vi "双通道示波器.vi"() -> ()   [LabVIEW 2022 SP3]
uses:
  <vilib>/Analysis/3filter.llb/Butterworth Filter (DBL).vi
  <vilib>/measure/matone.llb/Extract Single Tone Information 1 Chan.vi
  <vilib>/measure/NI_MABase.lvlib
  <vilib>/measure/NI_MAPro.lvlib
  <vilib>/Analysis/NI_AALBase.lvlib
panel:
  in  "选项卡控件":enum32{"基本参数", "滤波"}(tab)
  in  "CH0幅值单位调节":dbl(knob) scale=1.0..2.0
  in  "CH0幅值偏移":dbl(knob) scale=0.0..10.0
  in  "CH0":bool
  in  "CH1幅值单位调节":dbl(knob) scale=1.0..2.0
  in  "CH1幅值偏移":dbl(knob) scale=0.0..10.0
  in  "CH1":bool
  in  "CH1采样频率":i16(slide) scale=0.0..100.0
  in  "CH0采样频率":i16(slide) scale=0.0..100.0
  in  "CH0低截止频率":i16(slide) scale=0.0..5.0
  in  "CH0高截止频率":i16(slide) scale=0.0..5.0
  in  "CH0滤波器阶数":u8
  in  "CH1滤波器阶数":u8
  in  "CH1低截止频率":i16(slide) scale=0.0..5.0
  in  "CH1高截止频率":i16(slide) scale=0.0..10.0
  in  "CH1滤波器类型":u16(ring) items=["低通", "高通", "带通", "带阻"]
  in  "CH1滤波开关":bool
  in  "CH0滤波器类型":u16(ring) items=["低通", "高通", "带通", "带阻"]
  in  "CH0滤波开关":bool
  out "波形图":dbl[][](graph)
  out "CH1频率":dbl
  out "CH0频率":dbl
  out "CH0幅值":dbl
  out "CH1幅值":dbl
  out "CH1指示灯":bool
  out "CH0指示灯":bool
  in  "扫描频率":dbl(knob) scale=0.0..5.0
  in  "示波器开关":bool
  out "通道2指示灯":bool
  out "通道1指示灯":bool
  in  "信号发生器开关":bool
  in  "通道二开关":bool
  in  "通道一开关":bool
  in  "通道2自定义公式":string
  in  "通道2波形类型":u16(ring) items=["三角波", "正弦波", "自定义波形", "方波", "锯齿波"]
  out "通道2波形图表":waveform(dbl)(graph)
  in  "通道2偏移量":i64(knob) scale=-5.0..5.0
  in  "通道2标准差":dbl(knob) scale=0.0..1.0
  in  "通道2幅度":i64(knob) scale=0.0..10.0
  in  "通道2频率":dbl(knob) scale=0.0..1.0
  out "通道2波形信息":string
  out "通道1波形图表":waveform(dbl)(graph)
  out "通道1波形信息":string
  in  "通道1自定义公式":string
  in  "采样数":i64(slide) scale=1.0..5000.0
  in  "采样率":i64(slide) scale=150.0..1500.0
  in  "通道1偏移量":i64(knob) scale=-5.0..5.0
  in  "通道1标准差":dbl(knob) scale=0.0..1.0
  in  "通道1幅度":i64(knob) scale=0.0..10.0
  in  "通道1频率":dbl(knob) scale=0.0..1.0
  in  "通道1波形类型":u16(ring) items=["三角波", "正弦波", "自定义波形", "方波", "锯齿波"]
  # "信号发生器   MZ-0016"
  # "示波器  MZ-0016"
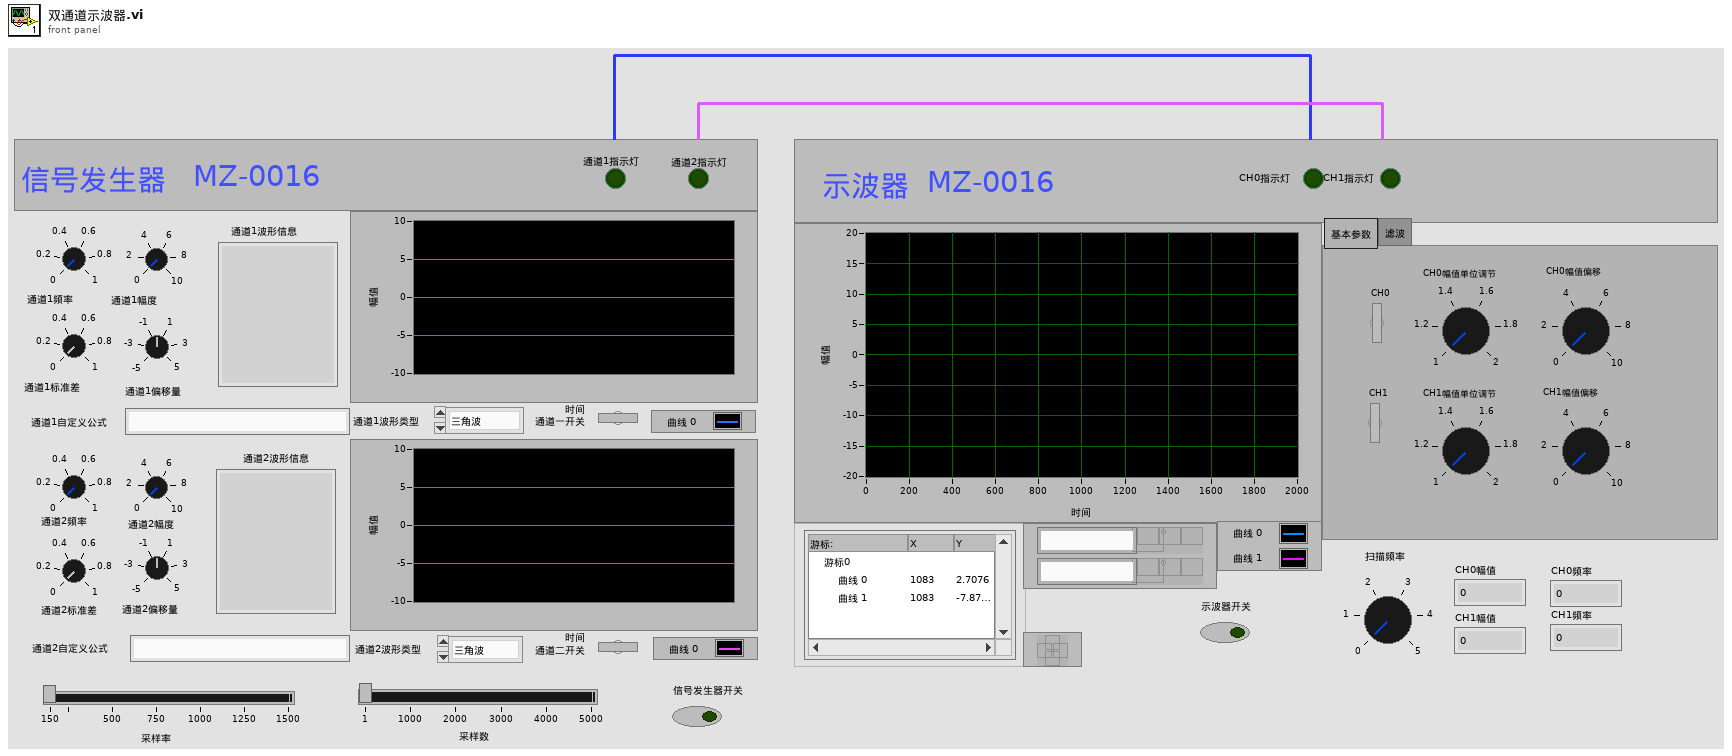
[diagram p1: front panel]
types:
  T1 = enum8{"Enabled", "Disabled", "Disabled and Grayed Out"}
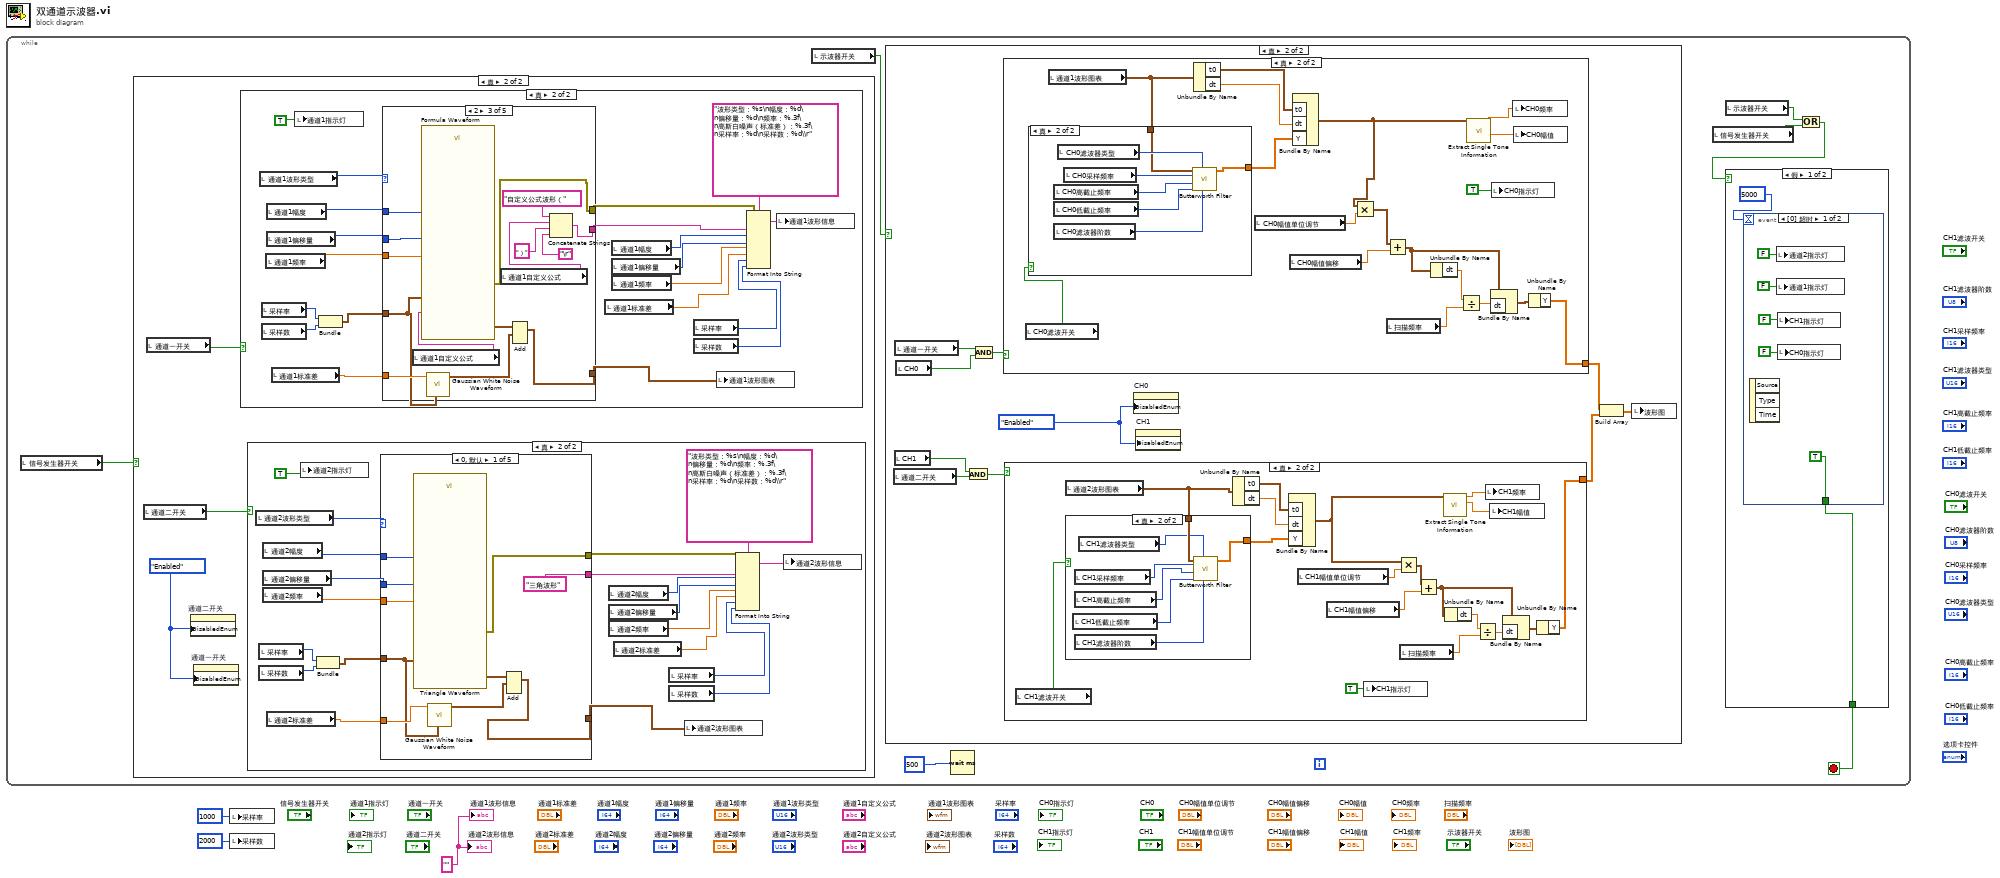
[diagram p0: block diagram]
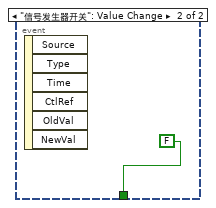
[diagram p2: hidden frame]
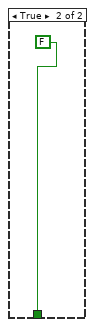
[diagram p3: hidden frame]
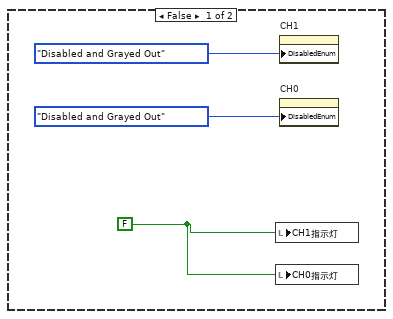
[diagram p4: hidden frame]
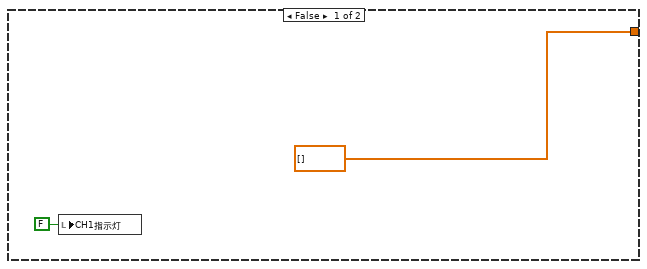
[diagram p5: hidden frame]
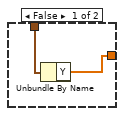
[diagram p6: hidden frame]
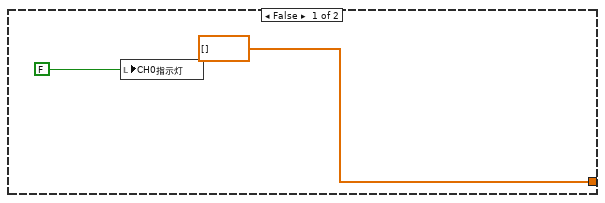
[diagram p7: hidden frame]
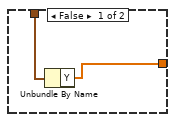
[diagram p8: hidden frame]
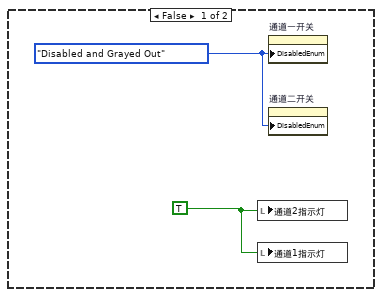
[diagram p9: hidden frame]
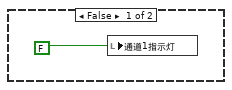
[diagram p10: hidden frame]
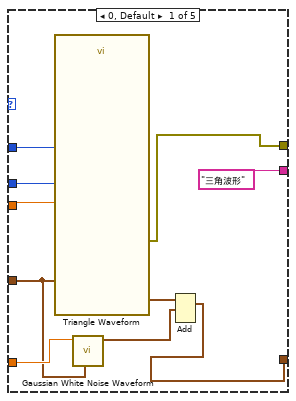
[diagram p11: hidden frame]
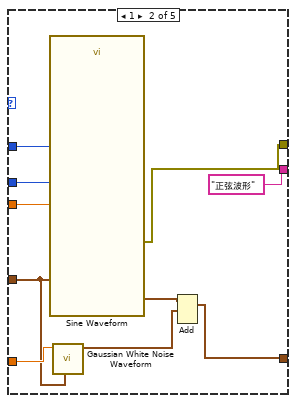
[diagram p12: hidden frame]
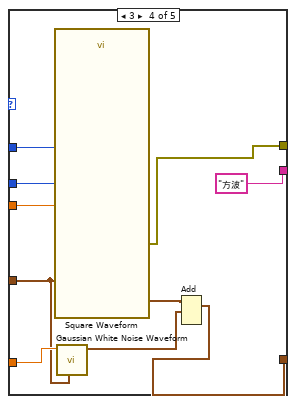
[diagram p13: hidden frame]
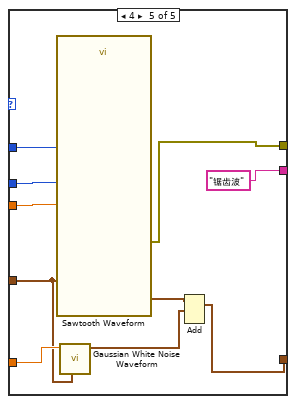
[diagram p14: hidden frame]
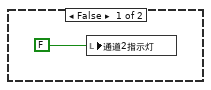
[diagram p15: hidden frame]
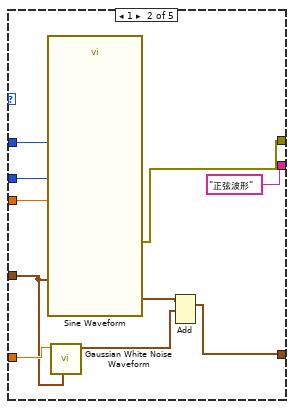
[diagram p16: hidden frame]
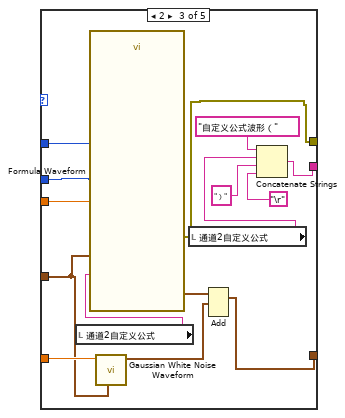
[diagram p17: hidden frame]
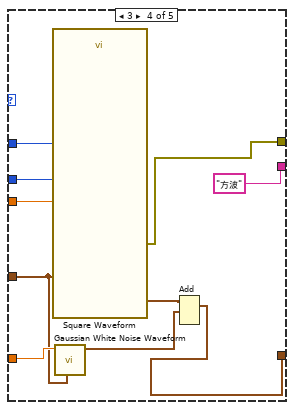
[diagram p18: hidden frame]
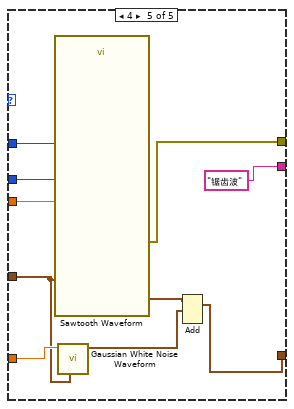
[diagram p19: hidden frame]
diagram:
  w3 = "" ("波形信息")
  n1 = while {
    stop <- w6 stop-if-true
    n2 = local read "信号发生器开关"() -> (w4:bool)
    n3 = case shown="真" w4 {
      frame False {
        w91 = T1."Disabled and Grayed Out" ("禁用")
        w92 = TRUE ("通道2指示灯")
        n4 = local write "通道2指示灯"(w92) -> ()
        n5 = local write "通道1指示灯"(w92) -> ()
        n6 = property on="通道一开关" class="Bool (严格)"("DisabledEnum"=w91) -> ()  [unwired: 2 in, 2 out]
        n7 = property on="通道二开关" class="Bool (严格)"("DisabledEnum"=w91) -> ()  [unwired: 2 in, 2 out]
      }
      frame True {
        w95 = T1."Enabled" ("禁用")
        n8 = local read "通道二开关"() -> (w93:bool)
        n9 = local read "通道一开关"() -> (w94:bool)
        n10 = property on="通道二开关" class="Bool (严格)"("DisabledEnum"=w95) -> ()  [unwired: 2 in, 2 out]
        n11 = property on="通道一开关" class="Bool (严格)"("DisabledEnum"=w95) -> ()  [unwired: 2 in, 2 out]
        n12 = case shown="真" w94 {
          frame False {
            n13 = local write "通道1指示灯"(FALSE ("通道1")) -> ()
          }
          frame True {
            n14 = local read "通道1波形类型"() -> (w116:u16)
            n15 = local read "采样率"() -> (w111:i64)
            n16 = local read "采样数"() -> (w110:i64)
            n17 = local read "通道1频率"() -> (w114:dbl)
            n18 = local read "通道1幅度"() -> (w112:i64)
            n19 = local read "通道1偏移量"() -> (w113:i64)
            n20 = local read "通道1标准差"() -> (w115:dbl)
            n21 = local write "通道1指示灯"(TRUE ("通道1")) -> ()
            n22 = Bundle("采样率"=w111, "采样数"=w110) -> (w109:cluster{"采样率":i64, "采样数":i64})  [unwired: 1 in]
            n23 = case shown="2" w116 {
              tunnel: w115 -> [w123 w133 w146 w155 w166]
              tunnel: w114 -> [w124 w134 w151 w158 w167]
              tunnel: w113 -> [w125 w135 w150 w157 w168]
              tunnel: w112 -> [w126 w136 w149 w156 w169]
              tunnel: w109 -> [w122 w132 w145 w154 w164]
              tunnel: [w119 w129 w139 w159 w165] -> w98
              tunnel: ["三角波形" "正弦波形" w138 "方波" "锯齿波"] -> w100
              tunnel: [w117 w127 w137 w152 w162] -> w99
              frame 0, Default {
                n24 = call <vilib>:"Triangle Waveform.vi"("offset"=w125, "sampling info"=w122, "amplitude"=w126, "frequency"=w124) -> ("error out"=w117:errorcluster, "signal out"=w121:waveform(dbl))  [unwired: 6 in]
                n25 = call <vilib>:"Gaussian White Noise Waveform.vi"("sampling info"=w122, "standard deviation"=w123) -> ("signal out"=w120:waveform(dbl))  [unwired: 8 in, 1 out]
                n26 = Add(1:w120, 2:w121) -> (0:w119:waveform(dbl))  [unwired: 1 in, 1 out]
              }
              frame 1 {
                n27 = call <vilib>:"Sine Waveform.vi"("offset"=w135, "sampling info"=w132, "amplitude"=w136, "frequency"=w134) -> ("error out"=w127:errorcluster, "signal out"=w131:waveform(dbl))  [unwired: 6 in]
                n28 = call <vilib>:"Gaussian White Noise Waveform.vi"("sampling info"=w132, "standard deviation"=w133) -> ("signal out"=w130:waveform(dbl))  [unwired: 8 in, 1 out]
                n29 = Add(1:w130, 2:w131) -> (0:w129:waveform(dbl))  [unwired: 1 in, 1 out]
              }
              frame 2 {
                n30 = local read "通道1自定义公式"() -> (w148:string)
                n31 = call <vilib>:"Formula Waveform.vi"("offset"=w150, "sampling info"=w145, "formula"=w148, "amplitude"=w149, "frequency"=w151) -> ("error out"=w137:errorcluster, "signal out"=w147:waveform(dbl))  [unwired: 5 in]
                n32 = call <vilib>:"Gaussian White Noise Waveform.vi"("sampling info"=w145, "standard deviation"=w146) -> ("signal out"=w144:waveform(dbl))  [unwired: 8 in, 1 out]
                n33 = local read "通道1自定义公式"() -> (w142:string)
                n34 = Add(1:w144, 2:w147) -> (0:w139:waveform(dbl))  [unwired: 1 in, 1 out]
                n35 = Concatenate Strings("自定义公式波形（", w142, "）" ("字符串"), "\r") -> (w138:string)
              }
              frame 3 {
                n36 = call <vilib>:"Square Waveform.vi"("offset"=w157, "sampling info"=w154, "amplitude"=w156, "frequency"=w158) -> ("error out"=w152:errorcluster, "signal out"=w161:waveform(dbl))  [unwired: 6 in]
                n37 = call <vilib>:"Gaussian White Noise Waveform.vi"("sampling info"=w154, "standard deviation"=w155) -> ("signal out"=w160:waveform(dbl))  [unwired: 8 in, 1 out]
                n38 = Add(1:w160, 2:w161) -> (0:w159:waveform(dbl))  [unwired: 1 in, 1 out]
              }
              frame 4 {
                n39 = call <vilib>:"Sawtooth Waveform.vi"("offset"=w168, "sampling info"=w164, "amplitude"=w169, "frequency"=w167) -> ("error out"=w162:errorcluster, "signal out"=w171:waveform(dbl))  [unwired: 6 in]
                n40 = call <vilib>:"Gaussian White Noise Waveform.vi"("sampling info"=w164, "standard deviation"=w166) -> ("signal out"=w170:waveform(dbl))  [unwired: 8 in, 1 out]
                n41 = Add(1:w170, 2:w171) -> (0:w165:waveform(dbl))  [unwired: 1 in, 1 out]
              }
            }
            n42 = local read "通道1标准差"() -> (w106:dbl)
            n43 = local read "通道1幅度"() -> (w103:i64)
            n44 = local read "通道1偏移量"() -> (w104:i64)
            n45 = local read "通道1频率"() -> (w105:dbl)
            n46 = local read "采样率"() -> (w107:i64)
            n47 = local read "采样数"() -> (w108:i64)
            n48 = local write "通道1波形图表"(w98) -> ()
            n49 = Format Into String(format string="波形类型：%s\n幅度：%d\n偏移量：%d\n频率：%.3f\n高斯白噪声（标准差）：%.3f\n采样率：%d\n采样数：%d\\r", error in=w99, w100, w103, w104, w105, w106, w107, w108) -> (resulting string=w101:string)  [unwired: 1 in, 1 out]
            n50 = local write "通道1波形信息"(w101) -> ()
          }
        }
        n51 = case shown="真" w93 {
          frame False {
            n52 = local write "通道2指示灯"(FALSE ("通道2")) -> ()
          }
          frame True {
            n53 = local read "通道2波形类型"() -> (w174:u16)
            n54 = local read "采样率"() -> (w179:i64)
            n55 = local read "采样数"() -> (w180:i64)
            n56 = local read "通道2幅度"() -> (w178:i64)
            n57 = local read "通道2偏移量"() -> (w177:i64)
            n58 = local read "通道2频率"() -> (w176:dbl)
            n59 = local read "通道2标准差"() -> (w175:dbl)
            n60 = local write "通道2指示灯"(TRUE ("通道2")) -> ()
            n61 = Bundle("采样率"=w179, "采样数"=w180) -> (w181:cluster{"采样率":i64, "采样数":i64})  [unwired: 1 in]
            n62 = case shown="0, 默认" w174 {
              tunnel: w175 -> [w199 w209 w222 w231 w242]
              tunnel: w176 -> [w200 w210 w227 w234 w243]
              tunnel: w177 -> [w201 w211 w226 w233 w244]
              tunnel: w178 -> [w202 w212 w225 w232 w245]
              tunnel: w181 -> [w198 w208 w221 w230 w240]
              tunnel: [w195 w205 w215 w235 w241] -> w192
              tunnel: ["三角波形" "正弦波形" w214 "方波" "锯齿波"] -> w190
              tunnel: [w193 w203 w213 w228 w238] -> w191
              frame 0, Default {
                n63 = call <vilib>:"Triangle Waveform.vi"("offset"=w201, "sampling info"=w198, "amplitude"=w202, "frequency"=w200) -> ("error out"=w193:errorcluster, "signal out"=w197:waveform(dbl))  [unwired: 6 in]
                n64 = call <vilib>:"Gaussian White Noise Waveform.vi"("sampling info"=w198, "standard deviation"=w199) -> ("signal out"=w196:waveform(dbl))  [unwired: 8 in, 1 out]
                n65 = Add(1:w196, 2:w197) -> (0:w195:waveform(dbl))  [unwired: 1 in, 1 out]
              }
              frame 1 {
                n66 = call <vilib>:"Sine Waveform.vi"("offset"=w211, "sampling info"=w208, "amplitude"=w212, "frequency"=w210) -> ("error out"=w203:errorcluster, "signal out"=w207:waveform(dbl))  [unwired: 6 in]
                n67 = call <vilib>:"Gaussian White Noise Waveform.vi"("sampling info"=w208, "standard deviation"=w209) -> ("signal out"=w206:waveform(dbl))  [unwired: 8 in, 1 out]
                n68 = Add(1:w206, 2:w207) -> (0:w205:waveform(dbl))  [unwired: 1 in, 1 out]
              }
              frame 2 {
                n69 = local read "通道2自定义公式"() -> (w224:string)
                n70 = call <vilib>:"Formula Waveform.vi"("offset"=w226, "sampling info"=w221, "formula"=w224, "amplitude"=w225, "frequency"=w227) -> ("error out"=w213:errorcluster, "signal out"=w223:waveform(dbl))  [unwired: 5 in]
                n71 = call <vilib>:"Gaussian White Noise Waveform.vi"("sampling info"=w221, "standard deviation"=w222) -> ("signal out"=w220:waveform(dbl))  [unwired: 8 in, 1 out]
                n72 = local read "通道2自定义公式"() -> (w218:string)
                n73 = Add(1:w220, 2:w223) -> (0:w215:waveform(dbl))  [unwired: 1 in, 1 out]
                n74 = Concatenate Strings("自定义公式波形（", w218, "）" ("字符串"), "\r") -> (w214:string)
              }
              frame 3 {
                n75 = call <vilib>:"Square Waveform.vi"("offset"=w233, "sampling info"=w230, "amplitude"=w232, "frequency"=w234) -> ("error out"=w228:errorcluster, "signal out"=w237:waveform(dbl))  [unwired: 6 in]
                n76 = call <vilib>:"Gaussian White Noise Waveform.vi"("sampling info"=w230, "standard deviation"=w231) -> ("signal out"=w236:waveform(dbl))  [unwired: 8 in, 1 out]
                n77 = Add(1:w236, 2:w237) -> (0:w235:waveform(dbl))  [unwired: 1 in, 1 out]
              }
              frame 4 {
                n78 = call <vilib>:"Sawtooth Waveform.vi"("offset"=w244, "sampling info"=w240, "amplitude"=w245, "frequency"=w243) -> ("error out"=w238:errorcluster, "signal out"=w247:waveform(dbl))  [unwired: 6 in]
                n79 = call <vilib>:"Gaussian White Noise Waveform.vi"("sampling info"=w240, "standard deviation"=w242) -> ("signal out"=w246:waveform(dbl))  [unwired: 8 in, 1 out]
                n80 = Add(1:w246, 2:w247) -> (0:w241:waveform(dbl))  [unwired: 1 in, 1 out]
              }
            }
            n81 = local read "通道2幅度"() -> (w187:i64)
            n82 = local read "通道2偏移量"() -> (w186:i64)
            n83 = local read "通道2频率"() -> (w185:dbl)
            n84 = local read "通道2标准差"() -> (w184:dbl)
            n85 = local read "采样率"() -> (w183:i64)
            n86 = local read "采样数"() -> (w182:i64)
            n87 = local write "通道2波形图表"(w192) -> ()
            n88 = Format Into String(format string="波形类型：%s\n幅度：%d\n偏移量：%d\n频率：%.3f\n高斯白噪声（标准差）：%.3f\n采样率：%d\n采样数：%d\\r", error in=w191, w190, w187, w186, w185, w184, w183, w182) -> (resulting string=w189:string)  [unwired: 1 in, 1 out]
            n89 = local write "通道2波形信息"(w189) -> ()
          }
        }
      }
    }
    n90 = local read "示波器开关"() -> (w9:bool)
    n91 = case shown="真" w9 {
      frame False {
        w20 = FALSE ("CH1指示灯")
        n92 = local write "CH1指示灯"(w20) -> ()
        n93 = local write "CH0指示灯"(w20) -> ()
        n94 = property on="CH1" class="Bool (严格)"("DisabledEnum"=T1."Disabled and Grayed Out" ("禁用")) -> ()  [unwired: 2 in, 2 out]
        n95 = property on="CH0" class="Bool (严格)"("DisabledEnum"=T1."Disabled and Grayed Out" ("禁用")) -> ()  [unwired: 2 in, 2 out]
      }
      frame True {
        w26 = T1."Enabled" ("禁用")
        n96 = local read "通道二开关"() -> (w30:bool)
        n97 = local read "CH1"() -> (w29:bool)
        n98 = local read "通道一开关"() -> (w32:bool)
        n99 = local read "CH0"() -> (w31:bool)
        n100 = And(x=w29, y=w30) -> (x .and. y?=w27:bool)
        n101 = And(x=w32, y=w31) -> (x .and. y?=w23:bool)
        n102 = case shown="真" w23 {
          tunnel: [dbl[] [] ("Y") w70] -> w25
          frame False {
            n103 = local write "CH0指示灯"(FALSE ("CH0指示灯")) -> ()
          }
          frame True {
            n104 = local read "CH0滤波开关"() -> (w64:bool)
            n105 = local read "通道1波形图表"() -> (w69:waveform(dbl))
            n106 = case shown="真" w64 {
              tunnel: w69 -> [w83 w89]
              tunnel: [w82 w84] -> w65
              frame False {
                n107 = Unbundle By Name(w83) -> ("Y"=w82:dbl[])
              }
              frame True {
                n108 = local read "CH0高截止频率"() -> (w87:i16)
                n109 = local read "CH0低截止频率"() -> (w86:i16)
                n110 = local read "CH0滤波器阶数"() -> (w85:u8)
                n111 = local read "CH0滤波器类型"() -> (w90:u16)
                n112 = local read "CH0采样频率"() -> (w88:i16)
                n113 = call-poly <vilib>:"Butterworth Filter.vi"("order"=w85, "filter type"=w90, "low cutoff freq: fl"=w86, "high cutoff freq: fh"=w87, "sampling freq: fs"=w88, "X"=w89) -> ("Filtered X"=w84:dbl[])  [unwired: 2 in, 1 out]
              }
            }
            n114 = Unbundle By Name(w69) -> ("t0"=w68:timestamp, "dt"=w67:dbl)
            n115 = local read "CH0幅值单位调节"() -> (w79:dbl)
            n116 = local read "CH0幅值偏移"() -> (w77:dbl)
            n117 = Bundle By Name("t0"=w68, "dt"=w67, "Y"=w65) -> (w66:waveform(dbl))  [unwired: 1 in]
            n118 = Multiply(x=w66, y=w79) -> (x*y=w78:waveform(dbl))
            n119 = Add(x=w78, y=w77) -> (x+y=w73:waveform(dbl))
            n120 = local read "扫描频率"() -> (w75:dbl)
            n121 = Unbundle By Name(w73) -> ("dt"=w76:dbl)
            n122 = Divide(x=w76, y=w75) -> (x/y=w74:dbl)
            n123 = call-poly <vilib>:"Extract Single Tone Information.vi"("time signal in"=w66) -> ("detected amplitude"=w80:dbl, "detected frequency"=w81:dbl)  [unwired: 5 in, 4 out]
            n124 = Bundle By Name(cluster=w73, "dt"=w74) -> (w72:waveform(dbl))
            n125 = local write "CH0指示灯"(TRUE ("CH0指示灯")) -> ()
            n126 = local write "CH0频率"(w81) -> ()
            n127 = local write "CH0幅值"(w80) -> ()
            n128 = Unbundle By Name(w72) -> ("Y"=w70:dbl[])
          }
        }
        n129 = case shown="真" w27 {
          tunnel: [dbl[] [] ("Y") w42] -> w24
          frame False {
            n130 = local write "CH1指示灯"(FALSE ("CH1指示灯")) -> ()
          }
          frame True {
            n131 = local read "CH1滤波开关"() -> (w35:bool)
            n132 = local read "通道2波形图表"() -> (w40:waveform(dbl))
            n133 = case shown="真" w35 {
              tunnel: w40 -> [w54 w61]
              tunnel: [w53 w60] -> w37
              frame False {
                n134 = Unbundle By Name(w54) -> ("Y"=w53:dbl[])
              }
              frame True {
                n135 = local read "CH1低截止频率"() -> (w56:i16)
                n136 = local read "CH1采样频率"() -> (w58:i16)
                n137 = local read "CH1高截止频率"() -> (w57:i16)
                n138 = local read "CH1滤波器阶数"() -> (w55:u8)
                n139 = local read "CH1滤波器类型"() -> (w59:u16)
                n140 = call-poly <vilib>:"Butterworth Filter.vi"("order"=w55, "filter type"=w59, "low cutoff freq: fl"=w56, "high cutoff freq: fh"=w57, "sampling freq: fs"=w58, "X"=w61) -> ("Filtered X"=w60:dbl[])  [unwired: 2 in, 1 out]
              }
            }
            n141 = Unbundle By Name(w40) -> ("t0"=w39:timestamp, "dt"=w38:dbl)
            n142 = Bundle By Name("t0"=w39, "dt"=w38, "Y"=w37) -> (w36:waveform(dbl))  [unwired: 1 in]
            n143 = local read "CH1幅值单位调节"() -> (w50:dbl)
            n144 = local read "CH1幅值偏移"() -> (w48:dbl)
            n145 = local write "CH1指示灯"(TRUE ("CH1指示灯")) -> ()
            n146 = Multiply(x=w36, y=w50) -> (x*y=w49:waveform(dbl))
            n147 = local read "扫描频率"() -> (w46:dbl)
            n148 = Add(x=w49, y=w48) -> (x+y=w44:waveform(dbl))
            n149 = call-poly <vilib>:"Extract Single Tone Information.vi"("time signal in"=w36) -> ("detected amplitude"=w51:dbl, "detected frequency"=w52:dbl)  [unwired: 5 in, 4 out]
            n150 = Unbundle By Name(w44) -> ("dt"=w47:dbl)
            n151 = Divide(x=w47, y=w46) -> (x/y=w45:dbl)
            n152 = local write "CH1频率"(w52) -> ()
            n153 = local write "CH1幅值"(w51) -> ()
            n154 = Bundle By Name(cluster=w44, "dt"=w45) -> (w43:waveform(dbl))
            n155 = Unbundle By Name(w43) -> ("Y"=w42:dbl[])
          }
        }
        n156 = property on="CH0" class="Bool (严格)"("DisabledEnum"=w26) -> ()  [unwired: 2 in, 2 out]
        n157 = property on="CH1" class="Bool (严格)"("DisabledEnum"=w26) -> ()  [unwired: 2 in, 2 out]
        n158 = Build Array(w25, w24) -> (w28:dbl[][])
        n159 = local write "波形图"(w28) -> ()
      }
    }
    n160 = Wait (ms)(milliseconds to wait=u32 500 ("毫秒计时值")) -> ()  [unwired: 1 out]
    n161 = local read "信号发生器开关"() -> (w7:bool)
    n162 = local read "示波器开关"() -> (w8:bool)
    n163 = Or(x=w8, y=w7) -> (x .or. y?=w5:bool)
    n164 = case shown="假" w5 {
      tunnel: [w12 FALSE] -> w6
      frame False {
        n165 = event shown="[0] 超时" {
          selector: _ -> [_ _]
          dyn-events: _ -> [_ _]
          timeout: 5000 -> [_ _]
          tunnel: [TRUE FALSE] -> w12
          event Timeout {
            n166 = event-data() -> ()  [unwired: 1 in, 3 out]
            n167 = local write "通道2指示灯"(FALSE ("通道2指示灯")) -> ()
            n168 = local write "通道1指示灯"(FALSE ("通道1指示灯")) -> ()
            n169 = local write "CH1指示灯"(FALSE ("CH1指示灯")) -> ()
            n170 = local write "CH0指示灯"(FALSE ("CH0指示灯")) -> ()
          }
          event "信号发生器开关": Value Change {
            n171 = event-data() -> ()  [unwired: 1 in, 6 out]
          }
        }
      }
      frame True {
      }
    }
  }
  n172 = local write "采样率"(i64 1000 ("采样率")) -> ()
  n173 = local write "采样数"(i64 2000 ("采样数")) -> ()
  "通道1波形信息" <- w3
  "通道2波形信息" <- w3
